vi "Neo Cortex.vi"() -> ()   [LabVIEW 2010]
uses:
  5.0-Global.vi
panel:
  out "Neo-C":bool
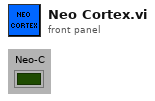
[diagram p1: front panel]
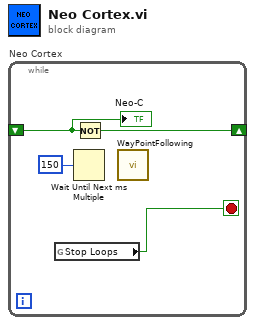
[diagram p0: block diagram]
diagram:
  n1 = while "Neo Cortex" {
    shift-right: [w3] -> _
    shift-left: _ -> [w2]
    stop <- w1 stop-if-true
    n2 = global read "5.0-Global.vi" "Stop Loops"() -> (w1:bool)
    n3 = Wait Until Next ms Multiple(millisecond multiple=u32 150 ("milliseconds to wait")) -> ()  [unwired: 1 out]
    n4 = Not(x=w2) -> (.not. x?=w3:bool)
    n5 = call "WayPointFollowing.vi"() -> ()  [unwired: 2 in]
    "Neo-C" <- w2
  }
